vi "NIDAQmx Logic.vi"(6 "initialize and close session behavior":T1=enum."Attach and Detach", 7 "connection type":T2, 8 "error in (no error)":errorcluster, 10 "Session Factory in":refnum<class "Session Factory.lvclass">, 11 "Measurement Configuration":T5) -> (0 "error out":errorcluster, 3 "Measurement Results":T4)   [LabVIEW 2021, in "NIDAQmxMeasurement.lvlib"]
doc: "This VI performs the DAQmx measurement."
uses:
  NIDAQmxMeasurement.lvlib
  Measurement Configuration.ctl
  Measurement Results.ctl
  <vilib>/Plug-In SDKs/Sessions/niDAQmx/Connection with Session.ctl
  <vilib>/Plug-In SDKs/Sessions/niDAQmx/Session Factory/Session Factory.lvclass
  <vilib>/Plug-In SDKs/Clients/Session Management V1/Session Reservation/Connection.ctl
  <vilib>/Plug-In SDKs/Clients/Session Management V1/Session Reservation/Initialize and Close Session Behavior.ctl
  <vilib>/Plug-In SDKs/Clients/Session Management V1/Session Reservation/Session Reservation.lvclass
  <vilib>/Plug-In SDKs/Sessions/niDAQmx/Session Management niDAQmx.lvlib
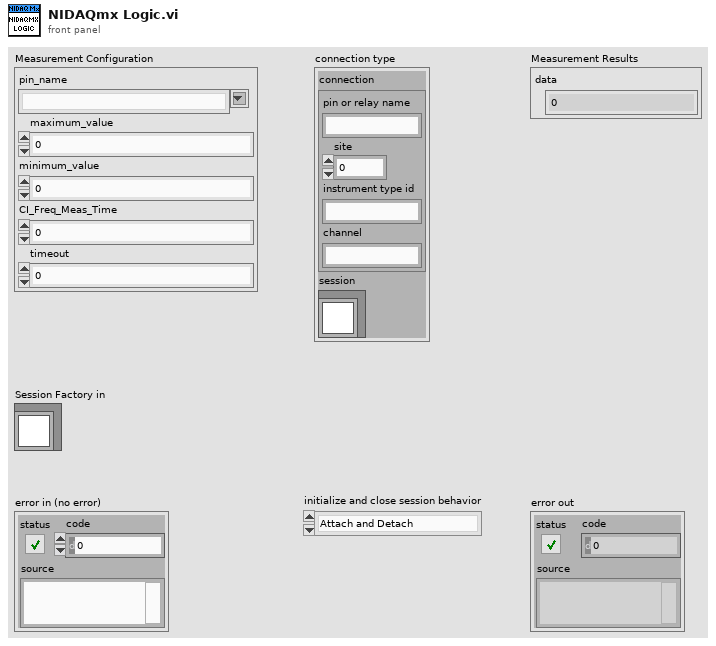
[diagram p1: front panel]
types:
  T1 = typedef "NI Session Management V1 Client.lvlib/Session Reservation.lvclass/Initialize and Close Session Behavior.ctl" = enum16{"Auto", "Initialize and Close", "Attach and Detach", "Initialize and Detach", "Attach and Close"}
  T2 = typedef "Session Management niDAQmx.lvlib/Connection with Session.ctl" = cluster{"connection":T3, "session":refnum<class "Session Factory.lvclass">}
  T3 = typedef "NI Session Management V1 Client.lvlib/Session Reservation.lvclass/Connection.ctl" = cluster{"pin or relay name":string, "site":i32, "instrument type id":string, "channel":string}
  T4 = typedef "NIDAQmxMeasurement.lvlib/Measurement Results.ctl" = cluster{"data":dbl}
  T5 = typedef "NIDAQmxMeasurement.lvlib/Measurement Configuration.ctl" = cluster{"pin_name":string, "maximum_value":dbl, "minimum_value":dbl, "CI_Freq_Meas_Time":dbl, "timeout":dbl}
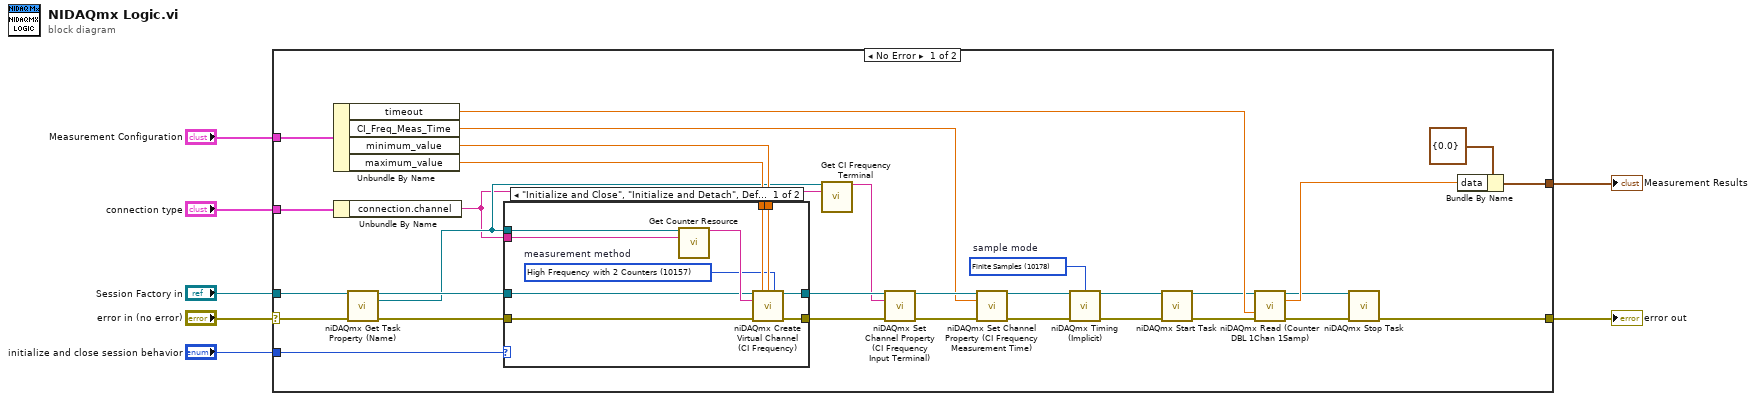
[diagram p0: block diagram]
diagram:
  n1 = case shown="No Error" "error in (no error)" {
    selector: "error in (no error)" -> [w33 w51]
    tunnel: "Measurement Configuration" -> [w38 _]
    tunnel: [w37 _] -> w6
    tunnel: [w35 w51] -> w5
    tunnel: "Session Factory in" -> [w32 _]
    tunnel: "connection type" -> [w34 _]
    tunnel: "initialize and close session behavior" -> [w8 _]
    frame No Error {
      w27 = 10178 items=["Finite Samples"=10178, "Continuous Samples"=10123, "Hardware Timed Single Point"=12522]  # sample mode
      n2 = Unbundle By Name(w38) -> ("timeout"=w30:dbl, "CI_Freq_Meas_Time"=w14:dbl, "minimum_value"=w28:dbl, "maximum_value"=w29:dbl)
      n3 = Unbundle By Name(w34) -> ("connection.channel"=w10:string)
      n4 = call <vilib>:"niDAQmx Get Task Property (Name).vi"("task in"=w32, "error in"=w33) -> ("task out"=w12:refnum<class "Session Factory.lvclass">, "Name"=w11:refnum<k21>, "error out"=w13:errorcluster)  [unwired: 11 in]
      n5 = case shown="\"Initialize and Close\", \"Initialize and Detach\", Default" w8 {
        tunnel: w29 -> [w47 _]
        tunnel: w28 -> [w46 _]
        tunnel: [w44 w50] -> w20
        tunnel: [w43 w49] -> w19
        tunnel: w13 -> [w42 w49]
        tunnel: w12 -> [w41 w50]
        tunnel: w11 -> [w40 _]
        tunnel: w10 -> [w39 _]
        frame "Initialize and Close", "Initialize and Detach", Default {
          w45 = 10157 items=["Low Frequency with 1 Counter"=10105, "High Frequency with 2 Counters"=10157, "Large Range with 2 Counters"=10205, "Dynamic Averaging"=16065]  # measurement method
          n6 = call "Get Counter Resource.vi"("Task Name"=w40, "channel"=w39) -> ("counter"=w48:tag)  [unwired: 13 in]
          n7 = call <vilib>:"niDAQmx Create Virtual Channel (CI Frequency).vi"("task in"=w41, "maximum value"=w47, "minimum value"=w46, "measurement method"=w45, "counter"=w48, "error in"=w42) -> ("task out"=w44:refnum<class "Session Factory.lvclass">, "error out"=w43:errorcluster)  [unwired: 8 in]
        }
        frame "Attach and Detach", "Attach and Close" {
        }
      }
      n8 = call "Get CI Frequency Terminal.vi"("Task Name"=w11, "channel"=w10) -> ("CI.Freq.Term"=w9:tag)  [unwired: 13 in]
      n9 = call <vilib>:"niDAQmx Set Channel Property (CI Frequency Input Terminal).vi"("task in"=w20, "CI.Freq.Term"=w9, "error in"=w19) -> ("task out"=w16:refnum<class "Session Factory.lvclass">, "error out"=w18:errorcluster)  [unwired: 11 in]
      n10 = call <vilib>:"niDAQmx Set Channel Property (CI Frequency Measurement Time).vi"("task in"=w16, "CI.Freq.MeasTime"=w14, "error in"=w18) -> ("task out"=w15:refnum<class "Session Factory.lvclass">, "error out"=w17:errorcluster)  [unwired: 11 in]
      n11 = call <vilib>:"niDAQmx Timing (Implicit).vi"("task in"=w15, "sample mode"=w27, "error in"=w17) -> ("task out"=w26:refnum<class "Session Factory.lvclass">, "error out"=w25:errorcluster)  [unwired: 11 in]
      n12 = call <vilib>:"niDAQmx Start Task.vi"("task in"=w26, "error in"=w25) -> ("task out"=w23:refnum<class "Session Factory.lvclass">, "error out"=w21:errorcluster)  [unwired: 12 in]
      n13 = call <vilib>:"niDAQmx Read (Counter DBL 1Chan 1Samp).vi"("task in"=w23, "timeout"=w30, "error in"=w21) -> ("task out"=w24:refnum<class "Session Factory.lvclass">, "data"=w31:dbl, "error out"=w22:errorcluster)  [unwired: 10 in]
      n14 = call <vilib>:"niDAQmx Stop Task.vi"("task in"=w24, "error in"=w22) -> ("error out"=w35:errorcluster)  [unwired: 12 in, 1 out]
      n15 = Bundle By Name(cluster=T4 {"data"=0.0} ("Measurement Results"), "data"=w31) -> (w37:T4)
    }
    frame Error {
    }
  }
  "Measurement Results" <- w6
  "error out" <- w5
